vi "Close Item Reference.vi"(8 "error in (no error)":errorcluster, 11 "VI in":refnum<class "VI.lvclass">) -> (0 "error out":errorcluster, 3 "VI out":refnum<class "VI.lvclass">)   [LabVIEW 2020, in "VI Properties Editor.lvlib" / "VI.lvclass"]
doc: "Closes the reference contained within the class data of <B>VI in</B>."
uses:
  VI.lvclass
  VI.lvclass/VI.ctl
panel:
  out "Application:All Libraries in Application Instance":string[](array[string])
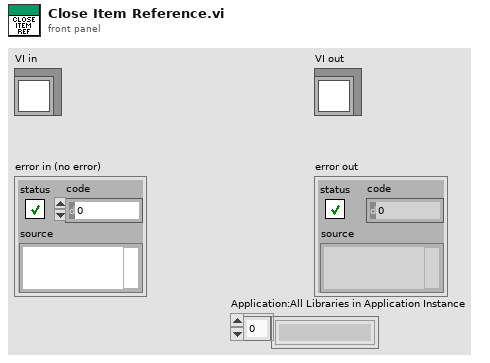
[diagram p1: front panel]
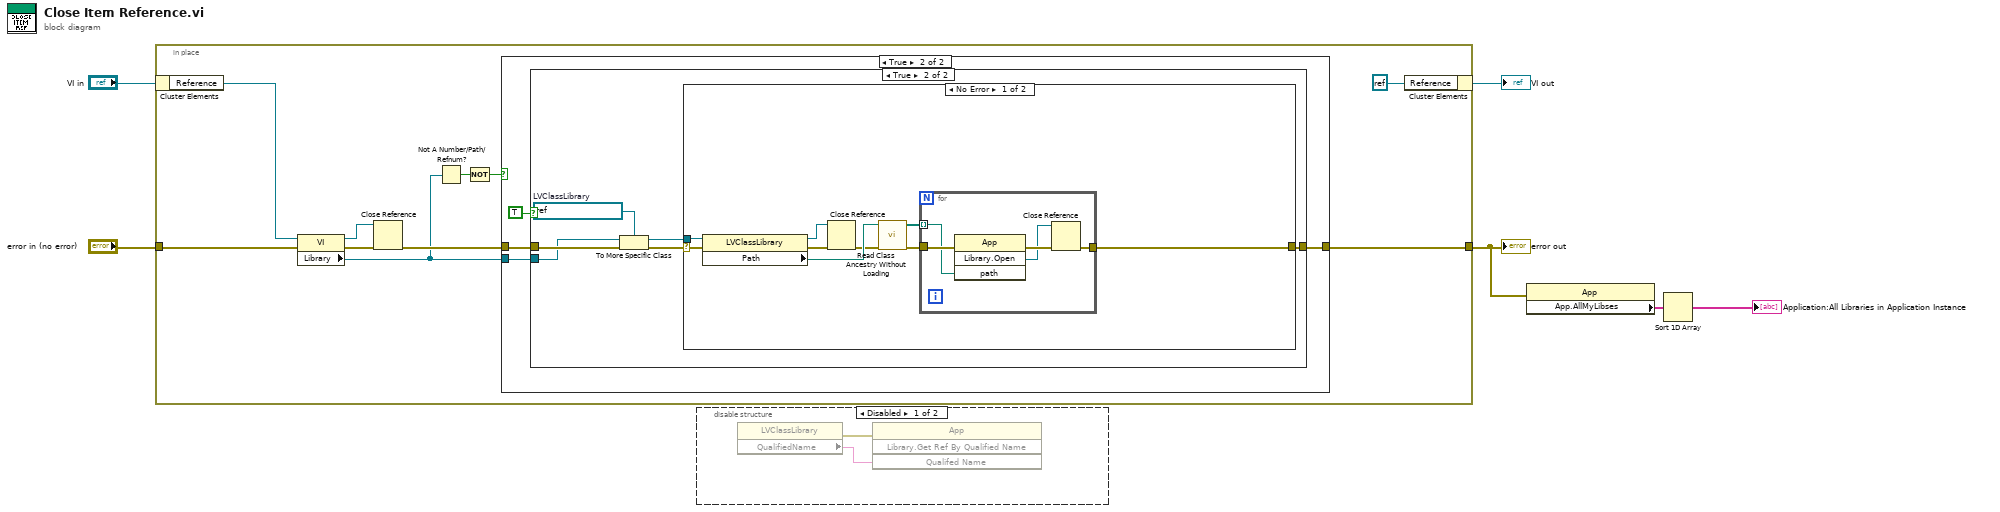
[diagram p0: block diagram]
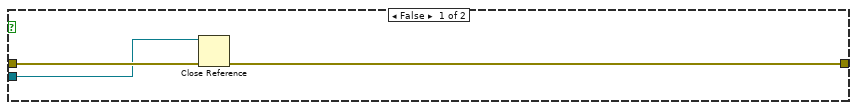
[diagram p4: hidden frame]
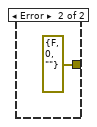
[diagram p5: hidden frame]
diagram:
  n1 = in-place {
    in-place-border: "error in (no error)" -> [w16]
    in-place-border: [w7] -> w2
    n2 = in-place-cluster #1("VI in") -> ("Reference"=w13:refnum<vi>)
    n3 = property class="VI"(reference=w13, error in=w16) -> (reference out=w12:refnum<vi>, error out=w14:errorcluster, "Library"=w8:refnum<vi>)
    n4 = Close Reference(reference=w12, error in (no error)=w14) -> (error out=w11:errorcluster)
    n5 = Not A Number/Path/Refnum?(number/path/refnum=w8) -> (NaN/Path/Refnum?=w10:bool)
    n6 = Not(x=w10) -> (.not. x?=w9:bool)
    n7 = case shown="True" w9 {
      tunnel: w11 -> [w17 w21]
      tunnel: w8 -> [_ w20]
      tunnel: [w17 w19] -> w7
      frame False {
      }
      frame True {
        n8 = case shown="True" TRUE {
          tunnel: w21 -> [w24 w30]
          tunnel: w20 -> [w22 w29]
          tunnel: [w23 w25] -> w19
          frame False {
            n9 = Close Reference(reference=w22, error in (no error)=w24) -> (error out=w23:errorcluster)
          }
          frame True {
            w28 = refnum<vi> refnum  # LVClassLibrary
            n10 = To More Specific Class(target class=w28, reference=w29, error in=w30) -> (specific class reference=w26:refnum<vi>, error out=w27:errorcluster)
            n11 = case shown="No Error" w27 {
              selector: w27 -> [w39 _]
              tunnel: w26 -> [w38 _]
              tunnel: [w31 errorcluster {"status"=FALSE, "code"=0, "source"=""} ("error out")] -> w25
              frame No Error {
                n12 = property class="LVClassLibrary"(reference=w38, error in=w39) -> (reference out=w32:refnum<vi>, error out=w37:errorcluster, "Path"=w36:path)
                n13 = Close Reference(reference=w32, error in (no error)=w37) -> (error out=w33:errorcluster)
                n14 = call <vilib>:"Read Class Ancestry Without Loading.vi"("error in (no error)"=w33, "LabVIEW Class Path"=w36) -> ("error out"=w35:errorcluster, "Class Ancestry"=w34:path[])  [unwired: 8 in]
                n15 = for {
                  tunnel: [w42] -> w31
                  tunnel: w35 -> [w41]
                  tunnel: w34 -> [w40] mode=indexing
                  n16 = invoke class="App" method="Library.Open"(error in=w41, "path"=w40) -> (error out=w44:errorcluster, "Open Library"=w43:refnum<vi>)  [unwired: 2 in, 2 out]
                  n17 = Close Reference(reference=w43, error in (no error)=w44) -> (error out=w42:errorcluster)
                }
              }
              frame Error {
              }
            }
          }
        }
      }
    }
    n18 = in-place-cluster #1("Reference"=refnum<k0> refnum) -> (→"VI out":refnum<class "VI.lvclass">)
  }
  "error out" <- w2
  n19 = disable-structure shown="Disabled" {
    frame Disabled {
      n20 = property class="LVClassLibrary"() -> (error out=w46:errorcluster, "QualifiedName"=w47:string)  [unwired: 2 in, 1 out]
      n21 = invoke class="App" method="Library.Get Ref By Qualified Name"(error in=w46, "Qualifed Name"=w47) -> ()  [unwired: 2 in, 4 out]
    }
    frame Enabled {
    }
  }
  n22 = property class="App"(error in=w2) -> ("App.AllMyLibses"=w3:string[])  [unwired: 1 in, 2 out]
  n23 = Sort 1D Array(array=w3) -> (sorted array=→"Application:All Libraries in Application Instance":string[])
